vi "Create Single element (Generic).vi"(7 "Type (Input)":T1, 8 "error in":errorcluster, 9 "type":string, 10 "name":string, 11 "Item Ref in":T2 format="%.0x") -> (0 "error out":errorcluster, 3 "Item Ref out":T2 format="%.0x")   [LabVIEW 2019, in "HLA Custom Device System Explorer.lvlib"]
uses:
  HLA Custom Device System Explorer.lvlib
  <vilib>/NI VeriStand/Custom Device API/Custom Device Item Ref.ctl
  <vilib>/NI VeriStand/Custom Device API/Custom Device Channel Type.ctl
  <vilib>/NI VeriStand/Custom Device API/Custom Device Channel.ctl
  Shared/Constants.vi
  <vilib>/NI VeriStand/Custom Device API/Custom Device API.lvlib
  Shared/HLA Custom Device Shared.lvlib
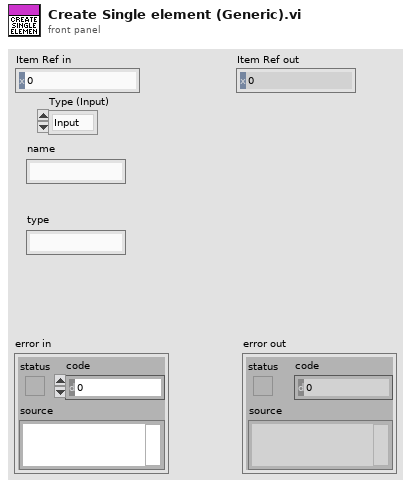
[diagram p1: front panel]
types:
  T1 = typedef "Custom Device API.lvlib/Custom Device Channel Type.ctl" = enum16{"Input", "Output"}
  T2 = typedef "Custom Device API.lvlib/Custom Device Item Ref.ctl" = u64
  T3 = typedef "Custom Device API.lvlib/Custom Device Channel.ctl" = cluster{"Type":T1, "Units":string, "Default Value":dbl, "Faultable":bool, "Scalable":bool}
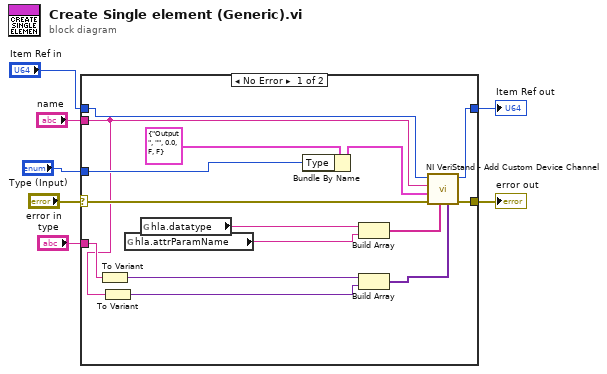
[diagram p0: block diagram]
diagram:
  n1 = case shown="No Error" "error in" {
    selector: "error in" -> [w21 w23]
    tunnel: [w20 w23] -> w6
    tunnel: [w18 w24] -> w5
    tunnel: "Item Ref in" -> [w19 w24]
    tunnel: "name" -> [w10 _]
    tunnel: "type" -> [w11 _]
    tunnel: "Type (Input)" -> [w16 _]
    frame No Error {
      n2 = To Variant(anything=w11) -> (Variant=w15:variant)
      n3 = To Variant(anything=w10) -> (Variant=w12:variant)
      n4 = global read "Constants.vi" "hla.attrParamName"() -> (w13:string)
      n5 = global read "Constants.vi" "hla.datatype"() -> (w14:string)
      n6 = Bundle By Name(cluster=T3 {"Type"=enum."Output", "Units"="", "Default Value"=0.0, "Faultable"=FALSE, "Scalable"=FALSE} ("Channel"), "Type"=w16) -> (w17:T3)
      n7 = Build Array(w14, w13) -> (w8:string[])
      n8 = Build Array(w15, w12) -> (w9:variant[])
      n9 = call <vilib>:"NI VeriStand - Add Custom Device Channel.vi"("Property Values"=w9, "Property names"=w8, "error in (no error)"=w21, "Channel"=w17, "Channel Name"=w10, "Parent Ref in"=w19) -> ("error out"=w20:errorcluster, "Parent Ref out"=w18:T2)  [unwired: 2 in, 2 out]
    }
    frame Error {
    }
  }
  "error out" <- w6
  "Item Ref out" <- w5
